vi "Demo test 2.vi"(0 "sub paenl vi path":path=path "D:/SLL Drona/Prototype/Issue 35 - Subpanel load Error/Subpanel VI.vi", 5 "vi path":path=path "D:/SLL Drona/Prototype/Issue 35 - Subpanel load Error/Demo VI.vi", 11 "error in":errorcluster) -> (3 "VI Ref same?":bool, 4 "VI Name":string, 15 "error out":errorcluster)   [LabVIEW 2016]
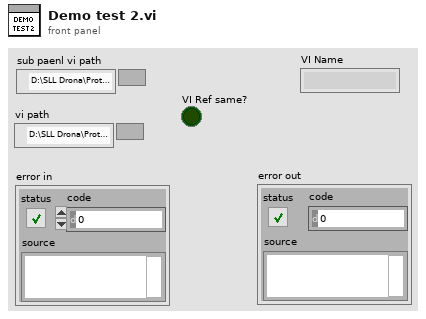
[diagram p1: front panel]
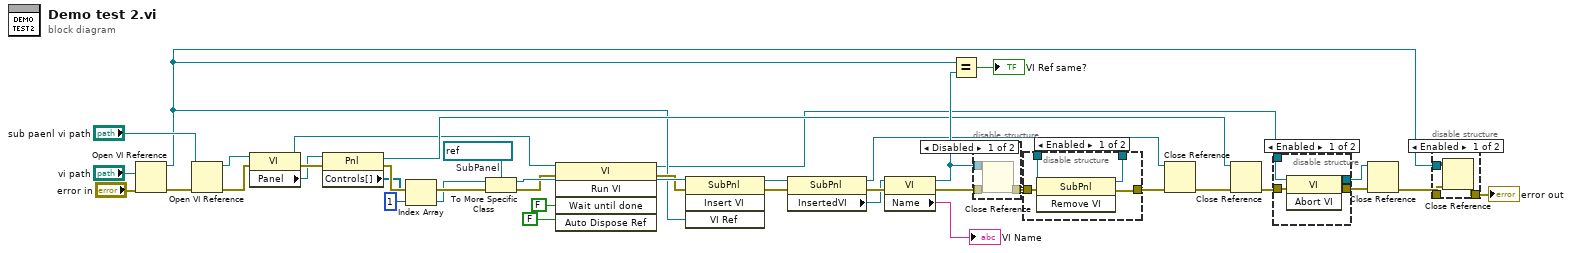
[diagram p0: block diagram]
diagram:
  w22 = refnum<vi> refnum  # SubPanel
  n1 = Open VI Reference(vi path="vi path", error in (no error)="error in") -> (vi reference=w8:refnum<vi>, error out=w31:errorcluster)  [unwired: 4 in]
  n2 = Open VI Reference(vi path="sub paenl vi path", error in (no error)=w31) -> (vi reference=w29:refnum<vi>, error out=w26:errorcluster)  [unwired: 4 in]
  n3 = property class="VI"(reference=w29, error in=w26) -> (reference out=w11:refnum<vi>, error out=w28:errorcluster, "Panel"=w27:refnum<vi>)
  n4 = property class="Pnl"(reference=w27, error in=w28) -> (reference out=w18:refnum<vi>, error out=w23:errorcluster, "Controls[]"=w21:refnum<vi>[])
  n5 = Index Array(array=w21, index=1) -> (element=w19:refnum<vi>)
  n6 = To More Specific Class(target class=w22, reference=w19, error in=w23) -> (specific class reference=w16:refnum<vi>, error out=w15:errorcluster)
  n7 = invoke class="VI" method="Run VI"(reference=w11, error in=w15, "Wait until done"=FALSE ("Wait Until Done"), "Auto Dispose Ref"=FALSE ("Auto Dispose Reference")) -> (reference out=w7:refnum<vi>, error out=w10:errorcluster)  [unwired: 1 in, 3 out]
  n8 = invoke class="SubPnl" method="Insert VI"(reference=w16, error in=w10, "VI Ref"=w8) -> (reference out=w25:refnum<vi>, error out=w24:errorcluster)  [unwired: 1 in, 2 out]
  n9 = property class="SubPnl"(reference=w25, error in=w24) -> (reference out=w13:refnum<vi>, error out=w38:errorcluster, "InsertedVI"=w35:refnum<vi>)
  n10 = property class="VI"(reference=w35, error in=w38) -> (reference out=w34:refnum<vi>, error out=w37:errorcluster, "Name"=→"VI Name":string)
  n11 = Equal?(x=w8, y=w34) -> (x = y?=→"VI Ref same?":bool)
  n12 = disable-structure shown="Disabled" {
    disable-tunnel: w34 -> [w43 _]
    disable-tunnel: w37 -> [w42 w44]
    disable-tunnel: [w41 w44] -> w32
    frame Disabled {
      n13 = Close Reference(reference=w43, error in (no error)=w42) -> (error out=w41:errorcluster)
    }
    frame Enabled {
    }
  }
  n14 = disable-structure shown="Enabled" {
    disable-tunnel: [w46 w49] -> w36
    disable-tunnel: w32 -> [w47 w49]
    disable-tunnel: w13 -> [w48 _]
    disable-tunnel: [w45 _] -> w12
    frame Enabled {
      n15 = invoke class="SubPnl" method="Remove VI"(reference=w48, error in=w47) -> (reference out=w45:refnum<vi>, error out=w46:errorcluster)  [unwired: 1 in, 1 out]
    }
    frame Disabled {
    }
  }
  n16 = Close Reference(reference=w12, error in (no error)=w36) -> (error out=w17:errorcluster)
  n17 = Close Reference(reference=w18, error in (no error)=w17) -> (error out=w2:errorcluster)
  n18 = disable-structure shown="Enabled" {
    disable-tunnel: w2 -> [w50 w55]
    disable-tunnel: [w53 w54] -> w4
    disable-tunnel: [w52 w55] -> w3
    disable-tunnel: w7 -> [w51 w54]
    frame Enabled {
      n19 = invoke class="VI" method="Abort VI"(reference=w51, error in=w50) -> (reference out=w53:refnum<vi>, error out=w52:errorcluster)  [unwired: 1 in, 1 out]
    }
    frame Disabled {
    }
  }
  n20 = Close Reference(reference=w4, error in (no error)=w3) -> (error out=w5:errorcluster)
  n21 = disable-structure shown="Enabled" {
    disable-tunnel: w5 -> [w58 w59]
    disable-tunnel: [w57 w59] -> w6
    disable-tunnel: w8 -> [w56 _]
    frame Enabled {
      n22 = Close Reference(reference=w56, error in (no error)=w58) -> (error out=w57:errorcluster)
    }
    frame Disabled {
    }
  }
  "error out" <- w6
